vi "CompareResult.vi"(11 "MulticolumnListbox in":refnum<vi>) -> (2 "Result":bool, 3 "MulticolumnListbox out":refnum<vi>)   [LabVIEW 2013]
uses:
  Control/Buffer.vi
panel:
  out "ledc":bool
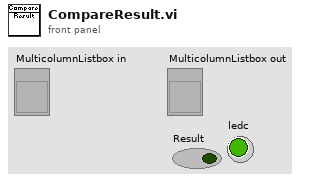
[diagram p1: front panel]
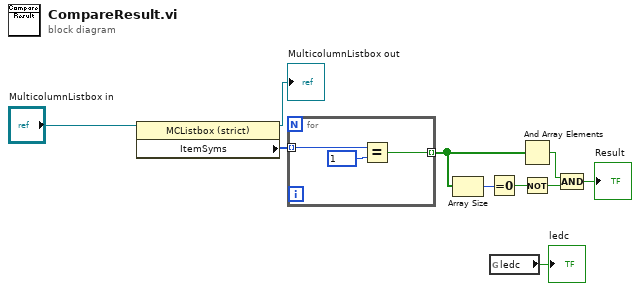
[diagram p0: block diagram]
diagram:
  n1 = property class="MCListbox (strict)"(reference="MulticolumnListbox in") -> (reference out=→"MulticolumnListbox out":refnum<vi>, "ItemSyms"=w3:i32[])  [unwired: 1 in, 1 out]
  n2 = for {
    tunnel: w3 -> [w13] mode=indexing
    tunnel: [w12] -> w5 mode=indexing
    n3 = Equal?(x=w13, y=1) -> (x = y?=w12:bool)
  }
  n4 = Array Size(array=w5) -> (size(s)=w6:i32)
  n5 = Equal To 0?(x=w6) -> (x = 0?=w7:bool)
  n6 = global read "Buffer.vi" "ledc"() -> (→"ledc":bool)
  n7 = And Array Elements(Boolean array=w5) -> (logical AND=w8:bool)
  n8 = Not(x=w7) -> (.not. x?=w9:bool)
  n9 = Compound Arithmetic op=AND(w8, w9) -> (→"Result":bool)
